vi "Ex 04-5 - CalcSOS.vi"() -> ()   [LabVIEW 2026]
uses:
  <instrlib>/MicroPulse/Public/Data/Datatypes/MP - data formatting.ctl
  <instrlib>/MicroPulse/Public/Data/Datatypes/MP - amplitude reporting mode.ctl
  <instrlib>/MicroPulse/Public/Data/Datatypes/MP - averaging.ctl
  <instrlib>/MicroPulse/Public/Data/Datatypes/MP - transmit parameters.ctl
  <instrlib>/MicroPulse/Public/Data/Datatypes/MP - pulser voltage.ctl
  <instrlib>/MicroPulse/Public/Data/Datatypes/MP - pulse damping.ctl
  <instrlib>/MicroPulse/Public/Data/Datatypes/MP - test parameters.ctl
  <instrlib>/MicroPulse/Public/Data/Datatypes/MP - receive parameters.ctl
  <instrlib>/MicroPulse/Public/Data/Datatypes/MP - display gate.ctl
  <instrlib>/MicroPulse/Public/Data/Datatypes/MP - waveform type.ctl
  <instrlib>/MicroPulse/Public/Data/Datatypes/MP - analogue filter.ctl
  <instrlib>/MicroPulse/Public/Data/Datatypes/MP - frequency filter.ctl
  <instrlib>/MicroPulse/Public/Data/Datatypes/MP - digital filtering.ctl
  <instrlib>/MicroPulse/Public/Data/Datatypes/MP - high pass filter.ctl
  <instrlib>/MicroPulse/Public/Data/Datatypes/MP - low pass filter.ctl
  <instrlib>/MicroPulse/Public/Data/Datatypes/TCP config.ctl
  <instrlib>/MicroPulse/Public/Data/Datatypes/MP - multi-gate inspection.ctl
  <instrlib>/MicroPulse/Public/Data/Datatypes/MP - multigate inspection gate parameters.ctl
  <instrlib>/MicroPulse/Public/Data/Datatypes/MP - hysteresis level.ctl
  <instrlib>/MicroPulse/Public/Data/Datatypes/MP - multigate mode.ctl
  <instrlib>/MicroPulse/Public/Data/Datatypes/MP - echo gate parameters.ctl
  <instrlib>/MicroPulse/Public/Data/Datatypes/MP - echo gate mode.ctl
  <instrlib>/MicroPulse/Public/Data/Datatypes/MP - data output format.ctl
  <instrlib>/MicroPulse/Public/Data/Datatypes/MP - instrument type.ctl
  <instrlib>/MicroPulse/Public/Data/Datatypes/MP - sample frequency.ctl
  <instrlib>/MicroPulse/MicroPulse_Driver.lvlib
panel:
  out "SOS":dbl[](array[numeric])=[5542.725173210162, 5600.9334889148195, 5587.892898719443] format="%#.2f m/s"
  in  "Sample thickness":dbl=12.0 format="%#_6f mm"
  out "Sample Frequency":T1=enum."100MHz"
  out "Instrument Type":T2=enum."Simulated Data"
  in  "Data Output Format":T3=enum."8-bit Mode" caption="[DOF]"
  in  "PRF":u16=50 caption="[PRF]" min=1 max=20000 step=100 format="%dHz"
  in  "Gate No.":i32=1 min=1 max=4
  out "peak data":cluster{"Time":dbl[], "Level":u16[]}={"Time"=[9.05], "Level"=[53]} {"Time" format="%_6g"}
  out "A-Scan + Peaks":cluster{"timebase":dbl[], "data":u16[]}[](graph)=[{"timebase"=array[5000 elements], "data"=array[5000 elements]}, {"timebase"=[9.05], "data"=[53]}, {"timebase"=[17.71], "data"=[65]}, {"timebase"=[26.28], "data"=[48]}, {"timebase"=[34.87], "data"=[49]}]
  in  "Echo Gate Mode":T4
  in  "Echo Gate Parameters":T5={"Start (us)"=15.0, "Length (us)"=20.0, "Threshold"=10, "Colour"=2731480} {"Threshold" min=10 max=4095 step=10; "Length (us)" min=0.0 max=96000.0 step=1.0; "Start (us)" min=0.0 max=64000.0 step=1.0}
  in  "Multi Gate Inspection":T6={"Gate 1"={"Start (us)"=8.0, "Length (us)"=4.0, "Threshold"=40, "Enabled?"=TRUE, "Max # Peaks"=8, "Hysteresis"=enum."6dB", "Mode"=enum."1st Threshold Crossing", "Inverted?"=FALSE, "Colour "=16716306}, "Gate 2"={"Start (us)"=16.0, "Length (us)"=4.0, "Threshold"=40, "Enabled?"=TRUE, "Max # Peaks"=8, "Hysteresis"=enum."6dB", "Mode"=enum."1st Threshold Crossing", "Inverted?"=FALSE, "Colour "=641024}, "Gate 3"={"Start (us)"=24.0, "Length (us)"=4.0, "Threshold"=40, "Enabled?"=TRUE, "Max # Peaks"=8, "Hysteresis"=enum."6dB", "Mode"=enum."1st Threshold Crossing", "Inverted?"=FALSE, "Colour "=4532}, "Gate 4"={"Start (us)"=34.0, "Length (us)"=4.0, "Threshold"=40, "Enabled?"=TRUE, "Max # Peaks"=8, "Hysteresis"=enum."6dB", "Mode"=enum."1st Threshold Crossing", "Inverted?"=FALSE, "Colour "=8978537}} {"Gate 4"."Max # Peaks" min=1 max=80 step=1; "Gate 4"."Threshold" min=10 step=10; "Gate 4"."Length (us)" min=0.0 max=96000.0 step=1.0; "Gate 4"."Start (us)" min=0.0 max=64000.0 step=1.0; "Gate 3"."Max # Peaks" min=1 max=80 step=1; "Gate 3"."Threshold" min=10 step=10; "Gate 3"."Length (us)" min=0.0 max=96000.0 step=1.0; "Gate 3"."Start (us)" min=0.0 max=64000.0 step=1.0; "Gate 2"."Max # Peaks" min=1 max=80 step=1; "Gate 2"."Threshold" min=10 step=10; "Gate 2"."Length (us)" min=0.0 max=96000.0 step=1.0; "Gate 2"."Start (us)" min=0.0 max=64000.0 step=1.0; "Gate 1"."Max # Peaks" min=1 max=80 step=1; "Gate 1"."Threshold" min=10 step=10; "Gate 1"."Length (us)" min=0.0 max=96000.0 step=1.0; "Gate 1"."Start (us)" min=0.0 max=64000.0 step=1.0}
  in  "Single Scan":bool
  in  "Stop Acquisition":bool
  in  "Start Acquisition":bool
  out "Command List":string="ENCM 2\r\nDOF 1\r\nPRF 50\r\nNUM 1\r\nTXN 1 1\r\nRXN 1 1\r\nAMP 1 32 \r\nPSV 1 50\r\nPDW 1 0 250\r\nGAT 1 0 5000\r\nDLY 1 0\r\nAWF 1 0\r\nGAN 1 137\r\nFRD 1 0 0\r\nETM 1 0\r\nGMT 1 1 800 1200\r\nHMS 1 1 2\r\nAMM 1 1 10\r\nPMG 1 1 8\r\nGIN 1 1 0\r\nUML 1 1 40\r\nAG.GMT_COL 1 1 FF1212\r\nGMT 1 2 1600 2000\r\nHMS 1 2 2\r\nAMM 1 2 10\r\nPMG 1 2 8\r\nGIN 1 2 0\r\nUML 1 2 40\r\nAG.GMT_COL 1 2 09C800\r\nGMT 1 3 2400 2800\r\nHMS 1 3 2\r\nAMM 1 3 10\r\nPMG 1 3 8\r\nGIN 1 3 0\r\nUML 1 3 40\r\nAG.GMT_COL 1 3 0011B4\r\nGMT 1 4 3400 3800\r\nHMS 1 4 2\r\nAMM 1 4 10\r\nPMG 1 4 8\r\nGIN 1 4 0\r\nUML 1 4 40\r\nAG.GMT_COL 1 4 890069\r"
  in  "QUIT":bool
  out "running average PRF":dbl=49.99631559070177 format="%0.2f"
  out "live error out":errorcluster={"status"=FALSE, "code"=56, "source"="TCP read timeout"}
  out "message count":i32=1
  out "System Messages":string="11:55:31\n------------------\nSTX 1 Completed\n------------------\nBuffer Cleared Successfully\n\n"
  in  "TCP config":T10={"Connection ID"=refnum, "IP address"="10.1.1.2", "host port"=1067, "OC timeout"=5000, "Read timeout"=2000, "Write timeout"=100} {"Write timeout" format="%dms"; "Read timeout" format="%dms"; "OC timeout" format="%dms"}
  in  "Receive Parameters":T11={"Display Gate"={"Start"=0.0, "Length"=50.0}, "Delay"=0.0, "Waveform Type"=enum."Rectified Signal", "Gain"=34.25, "Analogue Filtering"={"Bandpass"=enum."No change", "Smoothing"=1}, "Digital Filtering"={"High Pass Filter"=enum."None", "Low Pass Filter"=enum."None"}} {"Delay" format="%#_g us"; "Display Gate"."Length" min=0.0 max=64000.0 step=1.0 format="%#_g us"; "Display Gate"."Start" min=0.0 max=64000.0 step=1.0 format="%#_g us"; "Analogue Filtering"."Smoothing" min=1 max=11 step=1; "Gain" min=-6.0 max=70.0 step=0.25 format="%.2fdB"}
  in  "Test Parameters":T19={"Test No."=1, "Tx Channel"=1, "Rx Channel"=1} {"Rx Channel" min=1 max=1024; "Tx Channel" min=1 max=1024}
  in  "Transmit Parameters":T20={"Pulse Voltage"=enum."50V", "Pulse Shape"={"Damping"=enum."660W", "Width"=250}} {"Pulse Shape"."Width" min=16 max=1010 step=50 format="%.0fns"}
  in  "Data Formatting":T23={"Amplitude Mode"=enum."Peaks + Ascan for Multigate", "Averaging"=enum."None", "Coupling Level"=0} {"Coupling Level" max=4095 step=1}
  # "Example 04 - A-scan + Peaks Live Update\n\nSet all controls to the required values\nbefore running the VI.\n\nWhile running, test parameters may be changed."
  # "Place gates on the first four echos."
  # "Channels MUST be set BEFORE running"
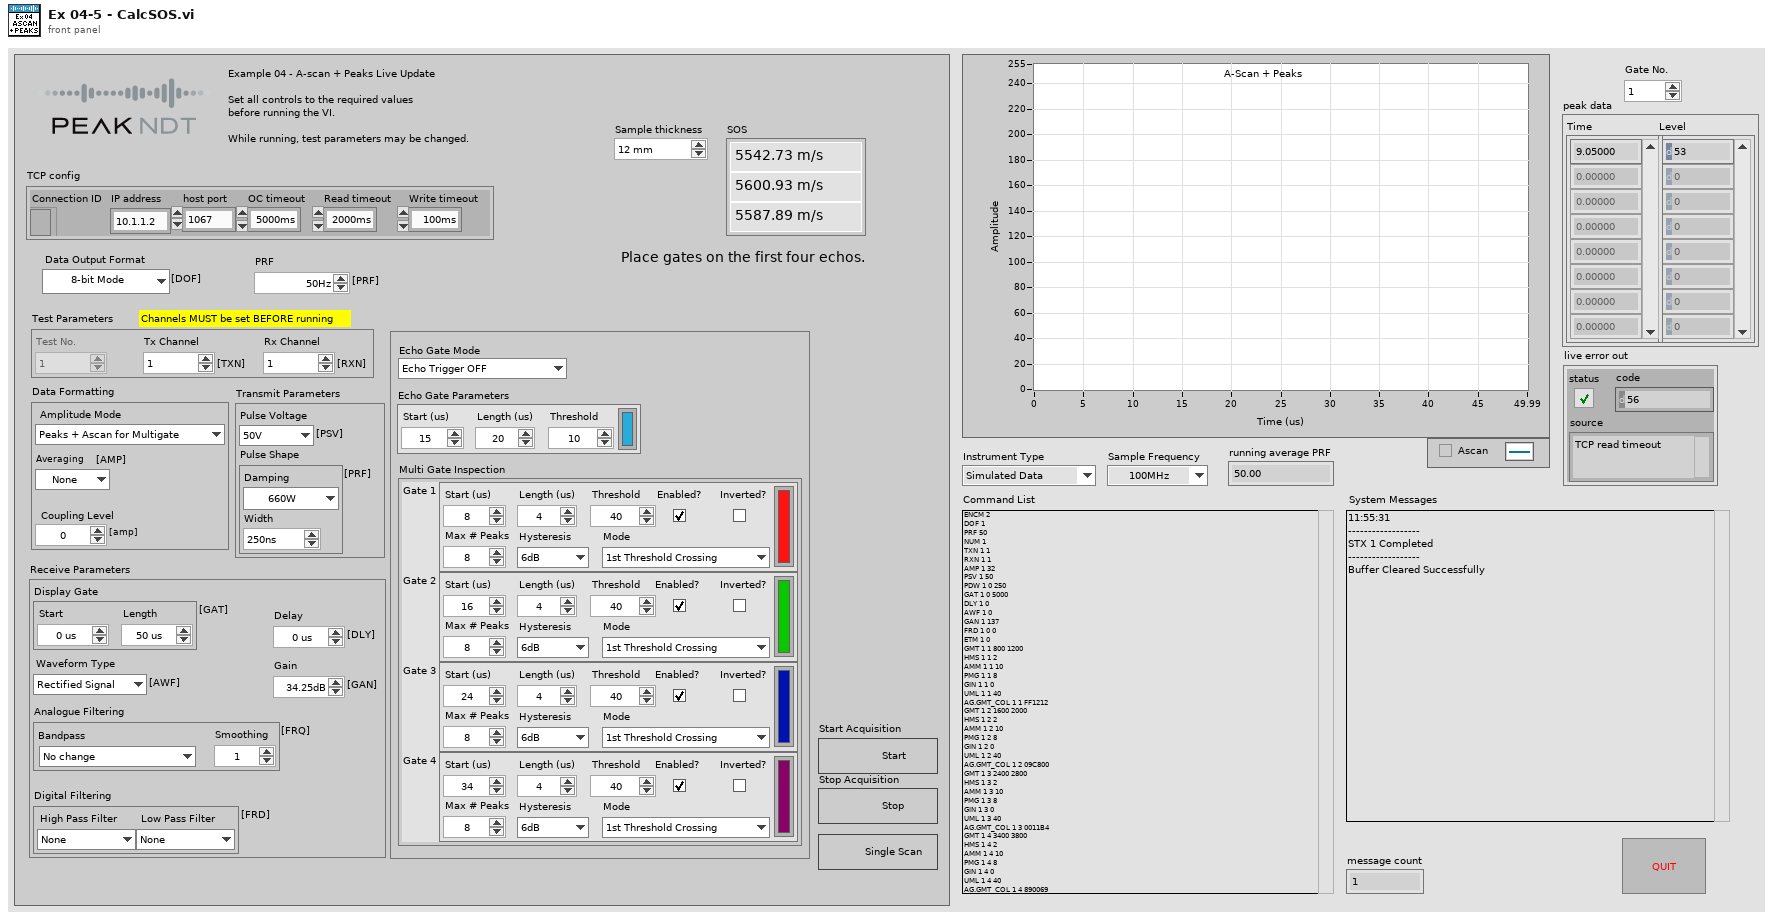
[diagram p1: front panel]
types:
  T1 = typedef "MicroPulse_Driver.lvlib/MP - sample frequency.ctl" = enum16{"Use Default", "200MHz (LT2 only)", "100MHz", "50MHz", "25MHz", "10MHz"}
  T2 = typedef "MicroPulse_Driver.lvlib/MP - instrument type.ctl" = enum16{"MicroPulse 5", "LT1", "LT2", "LTPA", "MPLT", "MicroPulse 6", "PipeScanner", "<MicroPulse>", "Micropulse 4", "Simulated Data"}
  T3 = typedef "MicroPulse_Driver.lvlib/MP - data output format.ctl" = enum16{"", "8-bit Mode", "10-bit Mode", "12-bit Mode", "16-bit Mode", "8-bit Log Mode", "12-bit Packed Mode"}
  T4 = typedef "MicroPulse_Driver.lvlib/MP - echo gate mode.ctl" = enum16{"Echo Trigger OFF", "Echo Gate Display Mode", "Echo Trigger ON", "Multi Gate or FMC Mode", "Reserved", "PA - Echo Trigger ON"}
  T5 = typedef "MicroPulse_Driver.lvlib/MP - echo gate parameters.ctl" = cluster{"Start (us)":dbl, "Length (us)":dbl, "Threshold":u16, "Colour":u32}
  T6 = typedef "MicroPulse_Driver.lvlib/MP - multi-gate inspection.ctl" = cluster{"Gate 1":T7, "Gate 2":T7, "Gate 3":T7, "Gate 4":T7}
  T7 = typedef "MicroPulse_Driver.lvlib/MP - multigate inspection gate parameters.ctl" = cluster{"Start (us)":dbl, "Length (us)":dbl, "Threshold":u16, "Enabled?":bool, "Max # Peaks":u16, "Hysteresis":T8, "Mode":T9, "Inverted?":bool, "Colour ":u32}
  T8 = typedef "MicroPulse_Driver.lvlib/MP - hysteresis level.ctl" = enum16{"None", "3dB", "6dB", "9dB", "12dB"}
  T9 = typedef "MicroPulse_Driver.lvlib/MP - multigate mode.ctl" = enum16{"1st Peak in Gate", "Largest Peak In Gate", "All Peaks In Gate", "1st Threshold Crossing"}
  T10 = typedef "MicroPulse_Driver.lvlib/TCP config.ctl" = cluster{"Connection ID":refnum<k5>, "IP address":string, "host port":u16, "OC timeout":i32, "Read timeout":i32, "Write timeout":i32}
  T11 = typedef "MicroPulse_Driver.lvlib/MP - receive parameters.ctl" = cluster{"Display Gate":T12, "Delay":dbl, "Waveform Type":T13, "Gain":dbl, "Analogue Filtering":T14, "Digital Filtering":T16}
  T12 = typedef "MicroPulse_Driver.lvlib/MP - display gate.ctl" = cluster{"Start":dbl, "Length":dbl}
  T13 = typedef "MicroPulse_Driver.lvlib/MP - waveform type.ctl" = enum16{"Rectified Signal", "RF Signal", "+Half Wave", "-Half Wave"}
  T14 = typedef "MicroPulse_Driver.lvlib/MP - analogue filter.ctl" = cluster{"Bandpass":T15, "Smoothing":u16}
  T15 = typedef "MicroPulse_Driver.lvlib/MP - frequency filter.ctl" = enum16{"No change", "1MHz Bandpass", "2MHz Bandpass", "4MHz Bandpass", "5MHz Bandpass", "10MHz Bandpass", "2.5-18MHz Broadband", "0.75-12MHz  Broadband", "0.5MHz Bandpass", "5MHz 2nd Order TOFD", "10MHz 2nd Order TOFD", "3.0-25MHz Broadband", "3.0-30MHz Broadband"}
  T16 = typedef "MicroPulse_Driver.lvlib/MP - digital filtering.ctl" = cluster{"High Pass Filter":T17, "Low Pass Filter":T18}
  T17 = typedef "MicroPulse_Driver.lvlib/MP - high pass filter.ctl" = enum16{"None", "0.7MHz", "1.5MHz", "4.0MHz", "7.5MHz", "10.0MHz", "User Defined"}
  T18 = typedef "MicroPulse_Driver.lvlib/MP - low pass filter.ctl" = enum16{"None", "1.8MHz", "3.0MHz", "6.0MHz", "8.0MHz", "12.0MHz", "User Defined"}
  T19 = typedef "MicroPulse_Driver.lvlib/MP - test parameters.ctl" = cluster{"Test No.":u32, "Tx Channel":u32, "Rx Channel":u32}
  T20 = typedef "MicroPulse_Driver.lvlib/MP - transmit parameters.ctl" = cluster{"Pulse Voltage":T21, "Pulse Shape":cluster{"Damping":T22, "Width":u32}}
  T21 = typedef "MicroPulse_Driver.lvlib/MP - pulser voltage.ctl" = enum16{"50V", "100V", "150V", "200V", "250V", "300V"}
  T22 = typedef "MicroPulse_Driver.lvlib/MP - pulse damping.ctl" = enum16{"660W", "458W", "220W", "149W", "102W", "82W", "63W", "51W"}
  T23 = typedef "MicroPulse_Driver.lvlib/MP - data formatting.ctl" = cluster{"Amplitude Mode":T24, "Averaging":T25, "Coupling Level":u32}
  T24 = typedef "MicroPulse_Driver.lvlib/MP - amplitude reporting mode.ctl" = enum16{"1st Peak in gate", "Maximum Peak in gate", "All Peaks", "Ascan Data", "1st Threshold Crossing Peak", "Ascan + Peaks", "All Peaks for Multigate", "Peaks + Ascan for Multigate", "Peaks + P_Ascan for Multigate", "Full Matrix Capture"}
  T25 = typedef "MicroPulse_Driver.lvlib/MP - averaging.ctl" = enum16{"None", "2", "4", "8", "16", "32", "64", "128", "256"}
  T26 = typedef "MicroPulse_Driver.lvlib/MP-Registry Data-Cluster.ctl" = cluster{"Instrument Type":T2, "Serial #":u64, "Sample Frequency":T1, "dt (us)":dbl, "DOF":T3, "Material Velocity":dbl, "Asynch Reads":T27, "NUM of Tests":u32, "System Details":T28, "Gates":T30[], "Encoders":T31[], "CMD LUT":variant, "Command List":string}
  T27 = typedef "MicroPulse_Driver.lvlib/MP - asynch read mode.ctl" = enum16{"Disabled", "Enabled"}
  T28 = typedef "MicroPulse_Driver.lvlib/MP - general system status.ctl" = cluster{"System Type":T2, "Serial No.":u64, "Channels":cluster{"Conv":u8, "PA":u16, "Extra":u32}, "Sample Frequency":cluster{"Default":u8, "Actual":u8}, "Software Versions":string, "Data Output Format":cluster{"Default":T3, "Actual":T3}, "Temperatures":cluster{"System":u8, "Processor":u8, "Slave Sys":u8, "Slave Proc":u8}, "Tx Buffer Size":u32, "System Error":string, "No. of Cards":u8, "DAC Gain":i16, "Uptimes":cluster{"since Power":u32, "since RSTS":u32, "since SRST":u32}, "Voltages":cluster{"Nominal":dbl, "Measured":dbl, "Difference":dbl}[], "Interface Cards":T29[]}
  T29 = typedef "MicroPulse_Driver.lvlib/MP - interface card status.ctl" = cluster{"Status":u8, "Map":u8, "Board - T":u8, "FPGA - T":u8, "PAIF Status":string, "Version":string}
  T30 = typedef "MicroPulse_Driver.lvlib/MP - Registry Gates.ctl" = cluster{"Display Gate":T12, "ETM Mode":T4, "Echo Gate":T5, "Insp Gates":T7[]}
  T31 = typedef "MicroPulse_Driver.lvlib/MP - encoder settings.ctl" = cluster{"Encoder Type":T32, "Counts/mm":u32, "Enable Termination?":bool, "Multiplier":u32, "Backlash Period (s)":dbl, "Encoder Filter":u32}
  T32 = typedef "MicroPulse_Driver.lvlib/MP - encoder type.ctl" = enum16{"Quadrature", "Step/Direction"}
  T33 = typedef "MicroPulse_Driver.lvlib/MP - scan data info.ctl" = cluster{"Message Header":u16, "Error Message":u16, "Test No.":u32, "Channel No.":u8, "Sweep No.":u32, "Gate No.":u32, "DOF":T3, "retain data":T34, "scan data":u16[], "scan length":i32, "scan index":i32, "peak data":cluster{"timebase":u16[], "data":u16[]}, "#peaks":i32, "PRF":dbl, "IP":cluster{"Axis No.":u8, "Location":u32, "MIP location":u32, "MIP?":bool}, "echo range":u16, "ETG":bool, "CAL 0 complete":bool, "Axis Positions":T35}
  T34 = typedef "MicroPulse_Driver.lvlib/MP - retain scan.ctl" = enum16{"None", "Ascan", "Peaks"}
  T35 = typedef "MicroPulse_Driver.lvlib/MP - axis positions (LLC).ctl" = cluster{"Axis 1":u32, "Axis 2":u32, "Axis 3":u32, "Axis 4":u32, "Status":u8}
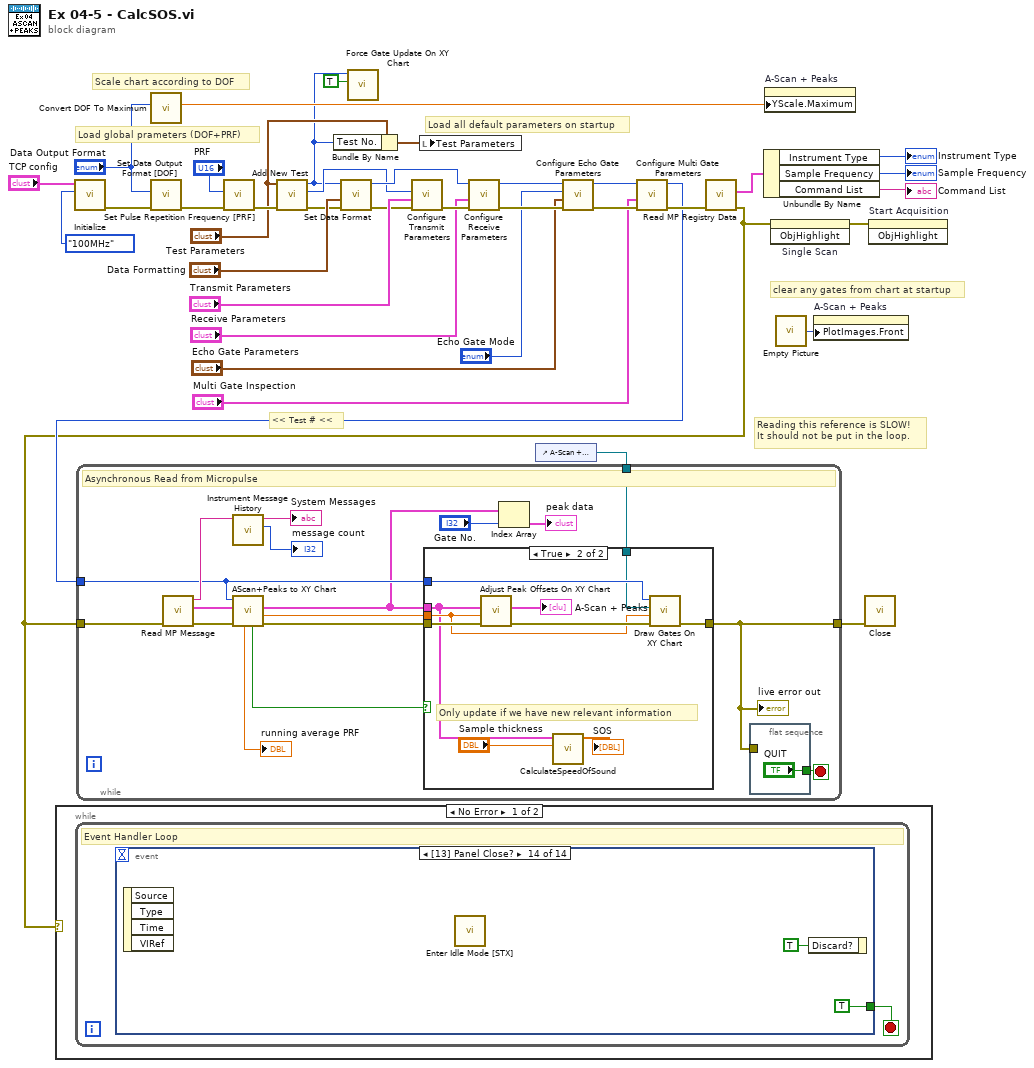
[diagram p0: block diagram]
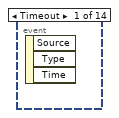
[diagram p2: hidden frame]
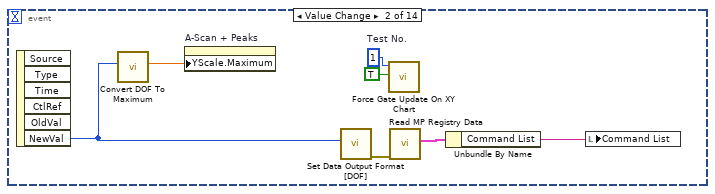
[diagram p3: hidden frame]
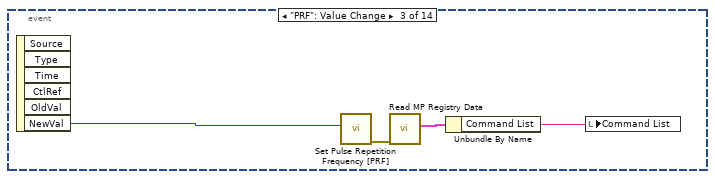
[diagram p4: hidden frame]
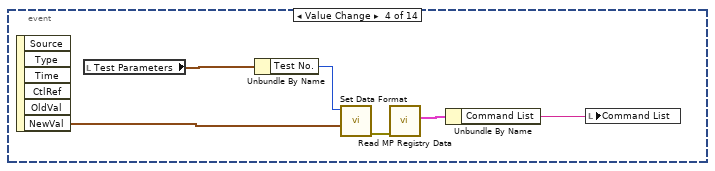
[diagram p5: hidden frame]
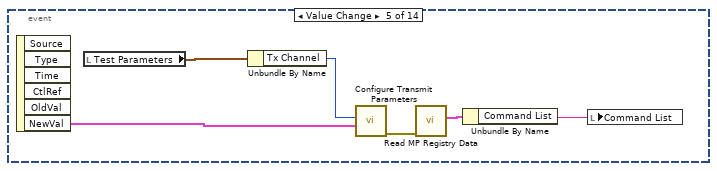
[diagram p6: hidden frame]
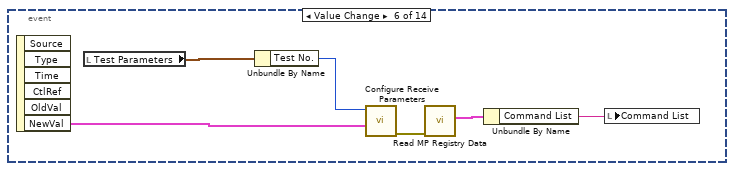
[diagram p7: hidden frame]
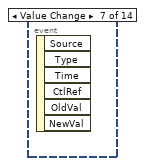
[diagram p8: hidden frame]
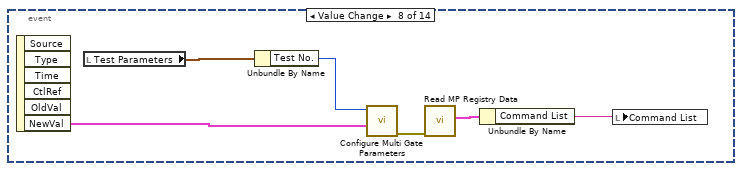
[diagram p9: hidden frame]
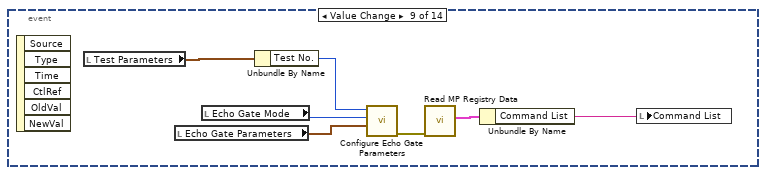
[diagram p10: hidden frame]
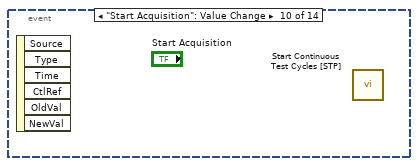
[diagram p11: hidden frame]
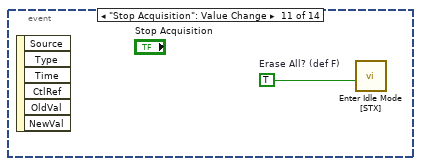
[diagram p12: hidden frame]
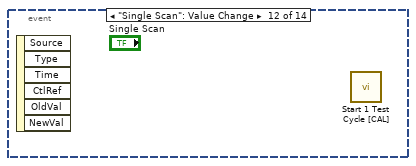
[diagram p13: hidden frame]
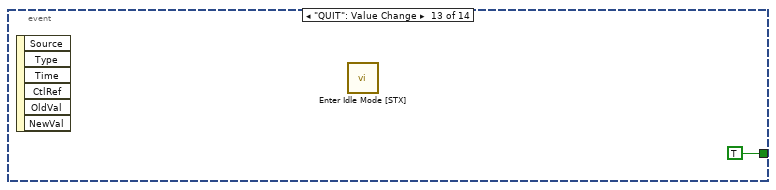
[diagram p14: hidden frame]
diagram:
  # "Scale chart according to DOF"
  # "Load global prameters (DOF+PRF)"
  # "Reading this reference is SLOW!\nIt should not be put in the loop."
  # "clear any gates from chart at startup"
  # "<< Test # <<"
  # "Load all default parameters on startup"
  n1 = call <instrlib>:"Initialize.vi"("Sample Frequency"=MP_-_sample_frequency."100MHz", "TCP config"="TCP config") -> ("error out"=w15:errorcluster)  [unwired: 8 in, 1 out]
  n2 = call <instrlib>:"Convert DOF To Maximum.vi"("Data Output Format"="Data Output Format") -> ("Data Maximum"=w5:dbl)  [unwired: 10 in]
  n3 = call <instrlib>:"Set Data Output Format [DOF].vi"("error in (no error)"=w15, "Mode"="Data Output Format") -> ("error out"=w14:errorcluster)  [unwired: 8 in, 1 out]
  n4 = call <instrlib>:"Set Pulse Repetition Frequency [PRF].vi"("error in (no error)"=w14, "Frequency (Hz)"="PRF") -> ("error out"=w13:errorcluster)  [unwired: 8 in, 1 out]
  n5 = call <instrlib>:"Add New Test.vi"("error in (no error)"=w13, "Test Parameters"="Test Parameters") -> ("error out"=w25:errorcluster, "Tx Channel out"=w10:u32, "Test No. out"=w4:u32)  [unwired: 6 in, 1 out]
  n6 = Bundle By Name(cluster="Test Parameters", "Test No."=w4) -> (w9:T19)
  n7 = call <instrlib>:"Set Data Format.vi"("error in (no error)"=w25, "Data Formatting"="Data Formatting", "Test No."=w4) -> ("error out"=w34:errorcluster, "Test No. out"=w27:u32)  [unwired: 6 in, 1 out]
  n8 = call <instrlib>:"Force Gate Update On XY Chart.vi"("Set?"=TRUE, "Test No."=w4) -> ()  [unwired: 7 in, 3 out]
  n9 = call <instrlib>:"Configure Transmit Parameters.vi"("error in (no error)"=w34, "Transmit Parameters"="Transmit Parameters", "Tx Channel"=w10) -> ("error out"=w35:errorcluster)  [unwired: 7 in, 1 out]
  n10 = local write "Test Parameters"(w9) -> ()
  n11 = call <instrlib>:"Configure Receive Parameters.vi"("error in (no error)"=w35, "Receive Parameters"="Receive Parameters", "Test No."=w27) -> ("error out"=w33:errorcluster, "Test No. out"=w28:u32)  [unwired: 6 in, 1 out]
  n12 = control-ref of="A-Scan + Peaks"() -> (w16:refnum<vi>)
  n13 = call <instrlib>:"Configure Echo Gate Parameters.vi"("error in (no error)"=w33, "Echo Gate Parameters"="Echo Gate Parameters", "Echo Trigger Mode"="Echo Gate Mode", "Test Number"=w28) -> ("error out"=w31:errorcluster, "Test Number Out"=w26:u32)  [unwired: 5 in, 1 out]
  n14 = call <instrlib>:"Configure Multi Gate Parameters.vi"("error in (no error)"=w31, "Multi Gate Inspection"="Multi Gate Inspection", "Test Number"=w26) -> ("error out"=w30:errorcluster, "Test Number out"=w24:u32)  [unwired: 6 in, 1 out]
  n15 = call <instrlib>:"Read MP Registry Data.vi"("error in (no error)"=w30) -> ("error out"=w18:errorcluster, "Micropulse Data"=w20:T26)  [unwired: 7 in, 2 out]
  n16 = case shown="No Error" w18 {
    frame No Error {
      n17 = while {
        stop <- w39 stop-if-true
        # "Event Handler Loop"
        n18 = event shown="[13] Panel Close?" {
          selector: _ -> [_ _ _ _ _ _ _ _ _ _ _ _ _ _]
          dyn-events: _ -> [_ _ _ _ _ _ _ _ _ _ _ _ _ _]
          timeout: _ -> [_ _ _ _ _ _ _ _ _ _ _ _ _ _]
          tunnel: [_ _ _ _ _ _ _ _ _ _ _ _ TRUE ("stop") TRUE ("stop")] -> w39
          event Timeout {
            n19 = event-data() -> ()  [unwired: 1 in, 3 out]
          }
          event Value Change {
            w41 = u32 1  # Test No.
            n20 = event-data() -> ("NewVal"=w42:T3)  [unwired: 1 in, 5 out]
            n21 = call <instrlib>:"Convert DOF To Maximum.vi"("Data Output Format"=w42) -> ("Data Maximum"=w43:dbl)  [unwired: 10 in]
            n22 = property on="A-Scan + Peaks" class="XYGraph (strict)"("YScale.Maximum"=w43) -> ()  [unwired: 2 in, 2 out]
            n23 = call <instrlib>:"Set Data Output Format [DOF].vi"("Mode"=w42) -> ("error out"=w46:errorcluster)  [unwired: 9 in, 1 out]
            n24 = call <instrlib>:"Force Gate Update On XY Chart.vi"("Set?"=TRUE, "Test No."=w41) -> ()  [unwired: 7 in, 3 out]
            n25 = call <instrlib>:"Read MP Registry Data.vi"("error in (no error)"=w46) -> ("Micropulse Data"=w45:T26)  [unwired: 7 in, 3 out]
            n26 = Unbundle By Name(w45) -> ("Command List"=w44:string)
            n27 = local write "Command List"(w44) -> ()
          }
          event "PRF": Value Change {
            n28 = event-data() -> ("NewVal"=w47:u16)  [unwired: 1 in, 5 out]
            n29 = call <instrlib>:"Set Pulse Repetition Frequency [PRF].vi"("Frequency (Hz)"=w47) -> ("error out"=w50:errorcluster)  [unwired: 9 in, 1 out]
            n30 = call <instrlib>:"Read MP Registry Data.vi"("error in (no error)"=w50) -> ("Micropulse Data"=w49:T26)  [unwired: 7 in, 3 out]
            n31 = Unbundle By Name(w49) -> ("Command List"=w48:string)
            n32 = local write "Command List"(w48) -> ()
          }
          event Value Change {
            n33 = event-data() -> ("NewVal"=w56:T23)  [unwired: 1 in, 5 out]
            n34 = local read "Test Parameters"() -> (w52:T19)
            n35 = Unbundle By Name(w52) -> ("Test No."=w51:u32)
            n36 = call <instrlib>:"Set Data Format.vi"("Data Formatting"=w56, "Test No."=w51) -> ("error out"=w55:errorcluster)  [unwired: 7 in, 2 out]
            n37 = call <instrlib>:"Read MP Registry Data.vi"("error in (no error)"=w55) -> ("Micropulse Data"=w54:T26)  [unwired: 7 in, 3 out]
            n38 = Unbundle By Name(w54) -> ("Command List"=w53:string)
            n39 = local write "Command List"(w53) -> ()
          }
          event Value Change {
            n40 = event-data() -> ("NewVal"=w61:T20)  [unwired: 1 in, 5 out]
            n41 = local read "Test Parameters"() -> (w62:T19)
            n42 = Unbundle By Name(w62) -> ("Tx Channel"=w60:u32)
            n43 = call <instrlib>:"Configure Transmit Parameters.vi"("Transmit Parameters"=w61, "Tx Channel"=w60) -> ("error out"=w58:errorcluster)  [unwired: 8 in, 1 out]
            n44 = call <instrlib>:"Read MP Registry Data.vi"("error in (no error)"=w58) -> ("Micropulse Data"=w59:T26)  [unwired: 7 in, 3 out]
            n45 = Unbundle By Name(w59) -> ("Command List"=w57:string)
            n46 = local write "Command List"(w57) -> ()
          }
          event Value Change {
            n47 = event-data() -> ("NewVal"=w66:T11)  [unwired: 1 in, 5 out]
            n48 = local read "Test Parameters"() -> (w68:T19)
            n49 = Unbundle By Name(w68) -> ("Test No."=w67:u32)
            n50 = call <instrlib>:"Configure Receive Parameters.vi"("Receive Parameters"=w66, "Test No."=w67) -> ("error out"=w65:errorcluster)  [unwired: 7 in, 2 out]
            n51 = call <instrlib>:"Read MP Registry Data.vi"("error in (no error)"=w65) -> ("Micropulse Data"=w63:T26)  [unwired: 7 in, 3 out]
            n52 = Unbundle By Name(w63) -> ("Command List"=w64:string)
            n53 = local write "Command List"(w64) -> ()
          }
          event Value Change {
            n54 = event-data() -> ()  [unwired: 1 in, 6 out]
          }
          event Value Change {
            n55 = event-data() -> ("NewVal"=w72:T6)  [unwired: 1 in, 5 out]
            n56 = local read "Test Parameters"() -> (w74:T19)
            n57 = Unbundle By Name(w74) -> ("Test No."=w73:u32)
            n58 = call <instrlib>:"Configure Multi Gate Parameters.vi"("Multi Gate Inspection"=w72, "Test Number"=w73) -> ("error out"=w71:errorcluster)  [unwired: 7 in, 2 out]
            n59 = call <instrlib>:"Read MP Registry Data.vi"("error in (no error)"=w71) -> ("Micropulse Data"=w70:T26)  [unwired: 7 in, 3 out]
            n60 = Unbundle By Name(w70) -> ("Command List"=w69:string)
            n61 = local write "Command List"(w69) -> ()
          }
          event Value Change {
            n62 = event-data() -> ()  [unwired: 1 in, 6 out]
            n63 = local read "Test Parameters"() -> (w81:T19)
            n64 = local read "Echo Gate Parameters"() -> (w77:T5)
            n65 = local read "Echo Gate Mode"() -> (w78:T4)
            n66 = Unbundle By Name(w81) -> ("Test No."=w79:u32)
            n67 = call <instrlib>:"Configure Echo Gate Parameters.vi"("Echo Gate Parameters"=w77, "Echo Trigger Mode"=w78, "Test Number"=w79) -> ("error out"=w80:errorcluster)  [unwired: 6 in, 2 out]
            n68 = call <instrlib>:"Read MP Registry Data.vi"("error in (no error)"=w80) -> ("Micropulse Data"=w76:T26)  [unwired: 7 in, 3 out]
            n69 = Unbundle By Name(w76) -> ("Command List"=w75:string)
            n70 = local write "Command List"(w75) -> ()
          }
          event "Start Acquisition": Value Change {
            n71 = event-data() -> ()  [unwired: 1 in, 6 out]
            n72 = call <instrlib>:"Start Continuous Test Cycles [STP].vi"() -> ()  [unwired: 10 in, 2 out]
          }
          event "Stop Acquisition": Value Change {
            w82 = TRUE  # Erase All? (def F)
            n73 = event-data() -> ()  [unwired: 1 in, 6 out]
            n74 = call <instrlib>:"Enter Idle Mode [STX].vi"("Erase All? (def T)"=w82) -> ()  [unwired: 9 in, 2 out]
          }
          event "Single Scan": Value Change {
            n75 = event-data() -> ()  [unwired: 1 in, 6 out]
            n76 = call <instrlib>:"Start 1 Test Cycle [CAL].vi"() -> ()  [unwired: 10 in, 2 out]
          }
          event "QUIT": Value Change {
            n77 = event-data() -> ()  [unwired: 1 in, 6 out]
            n78 = call <instrlib>:"Enter Idle Mode [STX].vi"() -> ()  [unwired: 10 in, 2 out]
          }
          event Panel Close? {
            n79 = event-data() -> ()  [unwired: 1 in, 4 out]
            n80 = call <instrlib>:"Enter Idle Mode [STX].vi"() -> ()  [unwired: 10 in, 2 out]
            n81 = event-data("Discard?"=TRUE) -> ()  [unwired: 1 in, 1 out]
          }
        }
      }
    }
    frame Error {
    }
  }
  n82 = while {
    tunnel: w18 -> [w98]
    tunnel: w24 -> [w94]
    tunnel: w16 -> [w93]
    tunnel: [w86] -> w1
    stop <- w95 stop-if-true
    # "Asynchronous Read from Micropulse"
    n83 = call <instrlib>:"Read MP Message.vi"("error in (no error)"=w98) -> ("error out"=w99:errorcluster, "scan data info"=w97:T33, "Instrument Message"=w101:string)  [unwired: 6 in, 2 out]
    n84 = call <instrlib>:"Instrument Message History.vi"("Instrument Message"=w101) -> ("Message Count"=→"message count":i32, "Message History out"=→"System Messages":string)  [unwired: 9 in]
    n85 = call <instrlib>:"AScan+Peaks to XY Chart.vi"("error in (no error)"=w99, "scan data info"=w97, "Test No."=w94) -> ("error out"=w96:errorcluster, "Echo Range (us)"=w92:dbl, "AScan+Peaks"=w87:cluster{"timebase":dbl[], "data":u16[]}[], "Update Indicators?"=w90:bool, "Running Average PRF"=→"running average PRF":dbl)  [unwired: 3 in, 1 out]
    n86 = case shown="True" w90 {
      tunnel: w96 -> [w103 w113]
      tunnel: [w103 w112] -> w86
      tunnel: w87 -> [_ w104]
      tunnel: w94 -> [_ w110]
      tunnel: w93 -> [_ w109]
      tunnel: w92 -> [_ w108]
      frame False {
      }
      frame True {
        # "Only update if we have new relevant information"
        n87 = call <instrlib>:"Adjust Peak Offsets On XY Chart.vi"("error in (no error)"=w113, "Echo Range in"=w108, "AScan+Peaks in"=w104) -> ("error out"=w111:errorcluster, "AScan+Peaks out"=→"A-Scan + Peaks":cluster{"timebase":dbl[], "data":u16[]}[])  [unwired: 7 in]
        n88 = call <instrlib>:"CalculateSpeedOfSound.vi"("Sample thickness"="Sample thickness", "AScan+Peaks"=w104) -> ("SOS"=→"SOS":dbl[])  [unwired: 9 in]
        n89 = call <instrlib>:"Draw Gates On XY Chart.vi"("error in (no error)"=w111, "Echo Range"=w108, "XYGraph in"=w109, "Test No."=w110) -> ("error out"=w112:errorcluster)  [unwired: 7 in]
      }
    }
    "live error out" <- w86
    n90 = Index Array(array=w87, index="Gate No.") -> (element=→"peak data":cluster{"timebase":dbl[], "data":u16[]})
    n91 = flat-sequence {
      tunnel: ["QUIT"] -> w95
      tunnel: w86 -> [_]
      frame #0 {
      }
    }
  }
  n92 = Unbundle By Name(w20) -> ("Instrument Type"=→"Instrument Type":T2, "Sample Frequency"=→"Sample Frequency":T1, "Command List"=→"Command List":string)
  n93 = property on="A-Scan + Peaks" class="XYGraph (strict)"("YScale.Maximum"=w5) -> ()  [unwired: 2 in, 2 out]
  n94 = invoke on="Single Scan" class="Bool" method="ObjHighlight"(error in=w18) -> (error out=w17:errorcluster)  [unwired: 2 in, 2 out]
  n95 = call "Empty Picture"() -> ("empty picture"=w29:picture)
  n96 = property on="A-Scan + Peaks" class="XYGraph (strict)"("PlotImages.Front"=w29) -> ()  [unwired: 2 in, 2 out]
  n97 = call <instrlib>:"Close.vi"("error in (no error)"=w1) -> ()  [unwired: 9 in, 2 out]
  n98 = invoke on="Start Acquisition" class="Bool" method="ObjHighlight"(error in=w17) -> ()  [unwired: 2 in, 3 out]
